vi "TonePattern-Plot Mask.vi"(0 "Graph":refnum<vi>, 5 "Y-axis slider":refnum<vi>, 7 "Properties":T2, 9 "Data":T1, 11 "error in (no error)":errorcluster) -> (15 "error out":errorcluster)   [LabVIEW 2020]
uses:
  TonePattern-Properties.ctl
  TonePattern-Data.ctl
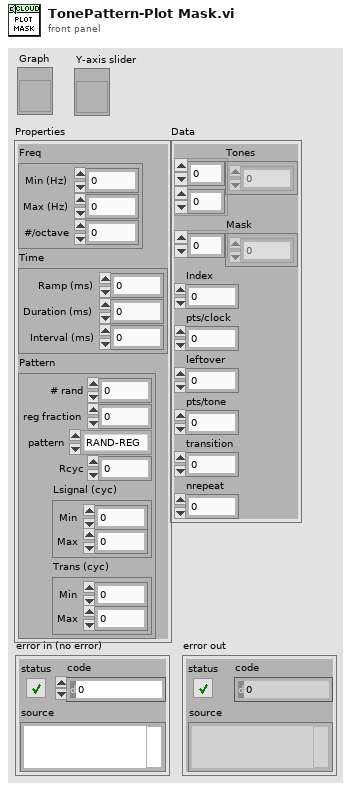
[diagram p1: front panel]
types:
  T1 = typedef "TonePattern-Data.ctl" = cluster{"Tones":dbl[][], "Mask":i32[], "Index":i32, "pts/clock":i32, "leftover":i32, "pts/tone":i32, "transition":i32, "nrepeat":i32}
  T2 = typedef "TonePattern-Properties.ctl" = cluster{"Freq":cluster{"Min (Hz)":dbl, "Max (Hz)":dbl, "#/octave":i32}, "Time":cluster{"Duration (ms)":dbl, "Interval (ms)":dbl, "Ramp (ms)":dbl}, "Pattern":cluster{"# rand":dbl, "reg fraction":dbl, "Rcyc":i32, "pattern":enum16{"RAND-REG", "REG-RAND", "RAND", "REG", "STEP", "CF"}, "Lsignal (cyc)":cluster{"Min":i32, "Max":i32}, "Trans (cyc)":cluster{"Min":i32, "Max":i32}}}
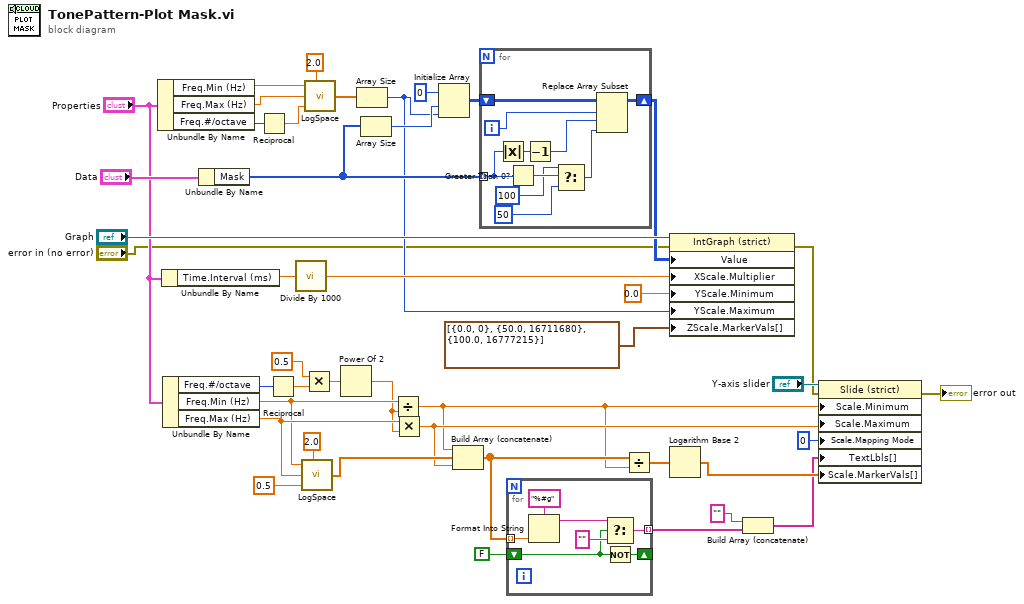
[diagram p0: block diagram]
diagram:
  n1 = Unbundle By Name("Properties") -> ("Freq.Min (Hz)"=w36:dbl, "Freq.Max (Hz)"=w35:dbl, "Freq.#/octave"=w34:i32)
  n2 = Unbundle By Name("Properties") -> ("Time.Interval (ms)"=w42:dbl)
  n3 = Unbundle By Name("Properties") -> ("Freq.#/octave"=w18:i32, "Freq.Min (Hz)"=w15:dbl, "Freq.Max (Hz)"=w19:dbl)
  n4 = Unbundle By Name("Data") -> ("Mask"=w38:i32[])
  n5 = Reciprocal(x=w34) -> (1/x=w33:dbl)
  n6 = Reciprocal(x=w18) -> (1/x=w17:dbl)
  n7 = call "Divide By 1000.vi"("X"=w42) -> ("X/1000"=w29:dbl)
  n8 = call "LogSpace.vi"("Start"=w15, "Base"=2.0, "Stop"=w19, "Step"=0.5) -> ("Array"=w20:dbl[])  [unwired: 2 in, 1 out]
  n9 = Multiply(x=0.5, y=w17) -> (x*y=w14:dbl)
  n10 = call "LogSpace.vi"("Start"=w36, "Base"=2.0, "Stop"=w35, "Step"=w33) -> ("Array"=w23:dbl[])  [unwired: 2 in, 1 out]
  n11 = Power Of 2(x=w14) -> (2^x=w12:dbl)
  n12 = Array Size(array=w23) -> (size(s)=w25:i32)
  n13 = Array Size(array=w38) -> (size(s)=w30:i32)
  n14 = Divide(x=w15, y=w12) -> (x/y=w6:dbl)
  n15 = Multiply(x=w19, y=w12) -> (x*y=w13:dbl)
  n16 = Initialize Array(0, w30, w25) -> (w40:i32[][])
  n17 = Build Array (concatenate)(w6, w20, w13) -> (w7:dbl[])
  n18 = for {
    tunnel: w38 -> [w48] mode=indexing
    shift-right: [w52] -> w31
    shift-left: w40 -> [w53]
    i -> [w51]
    n19 = Absolute Value(x=w48) -> (abs(x)=w50:i32)
    n20 = Greater Than 0?(x=w48) -> (x > 0?=w47:bool)
    n21 = Decrement(x=w50) -> (x-1=w49:i32)
    n22 = Select(t=100, s=w47, f=50) -> (s? t:f=w44:i32)
    n23 = Replace Array Subset(array=w53, new element=w44, index (row)=w51, index (col)=w49) -> (w52:i32[][])
  }
  n24 = for {
    tunnel: w7 -> [w60] mode=indexing
    shift-right: [w55] -> _
    shift-left: FALSE -> [w54]
    tunnel: [w58] -> w3 mode=indexing
    n25 = Format Into String(format string="%#g", w60) -> (resulting string=w57:string)  [unwired: 2 in, 1 out]
    n26 = Select(t=w57, s=w54, f="") -> (s? t:f=w58:string)
    n27 = Not(x=w54) -> (.not. x?=w55:bool)
  }
  n28 = Divide(x=w7, y=w6) -> (x/y=w5:dbl[])
  n29 = property class="IntGraph (strict)"(reference="Graph", error in="error in (no error)", "Value"=w31, "XScale.Multiplier"=w29, "YScale.Minimum"=0.0 ("Y Scale.Range:Minimum"), "YScale.Maximum"=w25, "ZScale.MarkerVals[]"=cluster{dbl, u32}[] [{0.0, 0}, {50.0, 16711680}, {100.0, 16777215}] ("Z Scale.Marker Values[]")) -> (error out=w9:errorcluster)  [unwired: 1 out]
  n30 = Logarithm Base 2(1:w5) -> (0:w4:dbl[])
  n31 = Build Array (concatenate)("", w3) -> (w2:string[])
  n32 = property class="Slide (strict)"(reference="Y-axis slider", error in=w9, "Scale.Minimum"=w6, "Scale.Maximum"=w13, "Scale.Mapping Mode"=u8 0, "TextLbls[]"=w2, "Scale.MarkerVals[]"=w4) -> (error out=→"error out":errorcluster)  [unwired: 1 out]
